vi "numpy_fft_fftfreq.vi"() -> ()   [LabVIEW 2020]
panel:
  out "n*d":fxp<+,32,16>
  out "val":fxp<+,64,48>
  out "f":fxp<+/-,32,16>[](array[numeric])
  out "Numeric":i32
  in  "s (sample rate)":fxp<+,16,16>
  out "p 2":fxp<+/-,32,32>[](array[numeric])
  out "output array":fxp<+/-,32,32>[](array[numeric])
  out "p1":fxp<+/-,32,32>[](array[numeric])
  out "N":fxp<+/-,18,17>
  in  "n":fxp<+,16,16>
  # "n=512"
  # "s=51200"
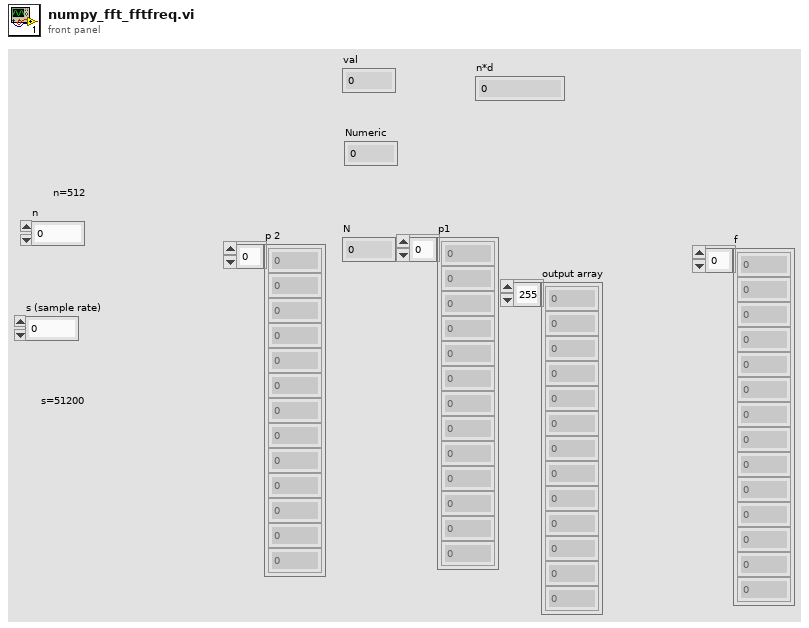
[diagram p1: front panel]
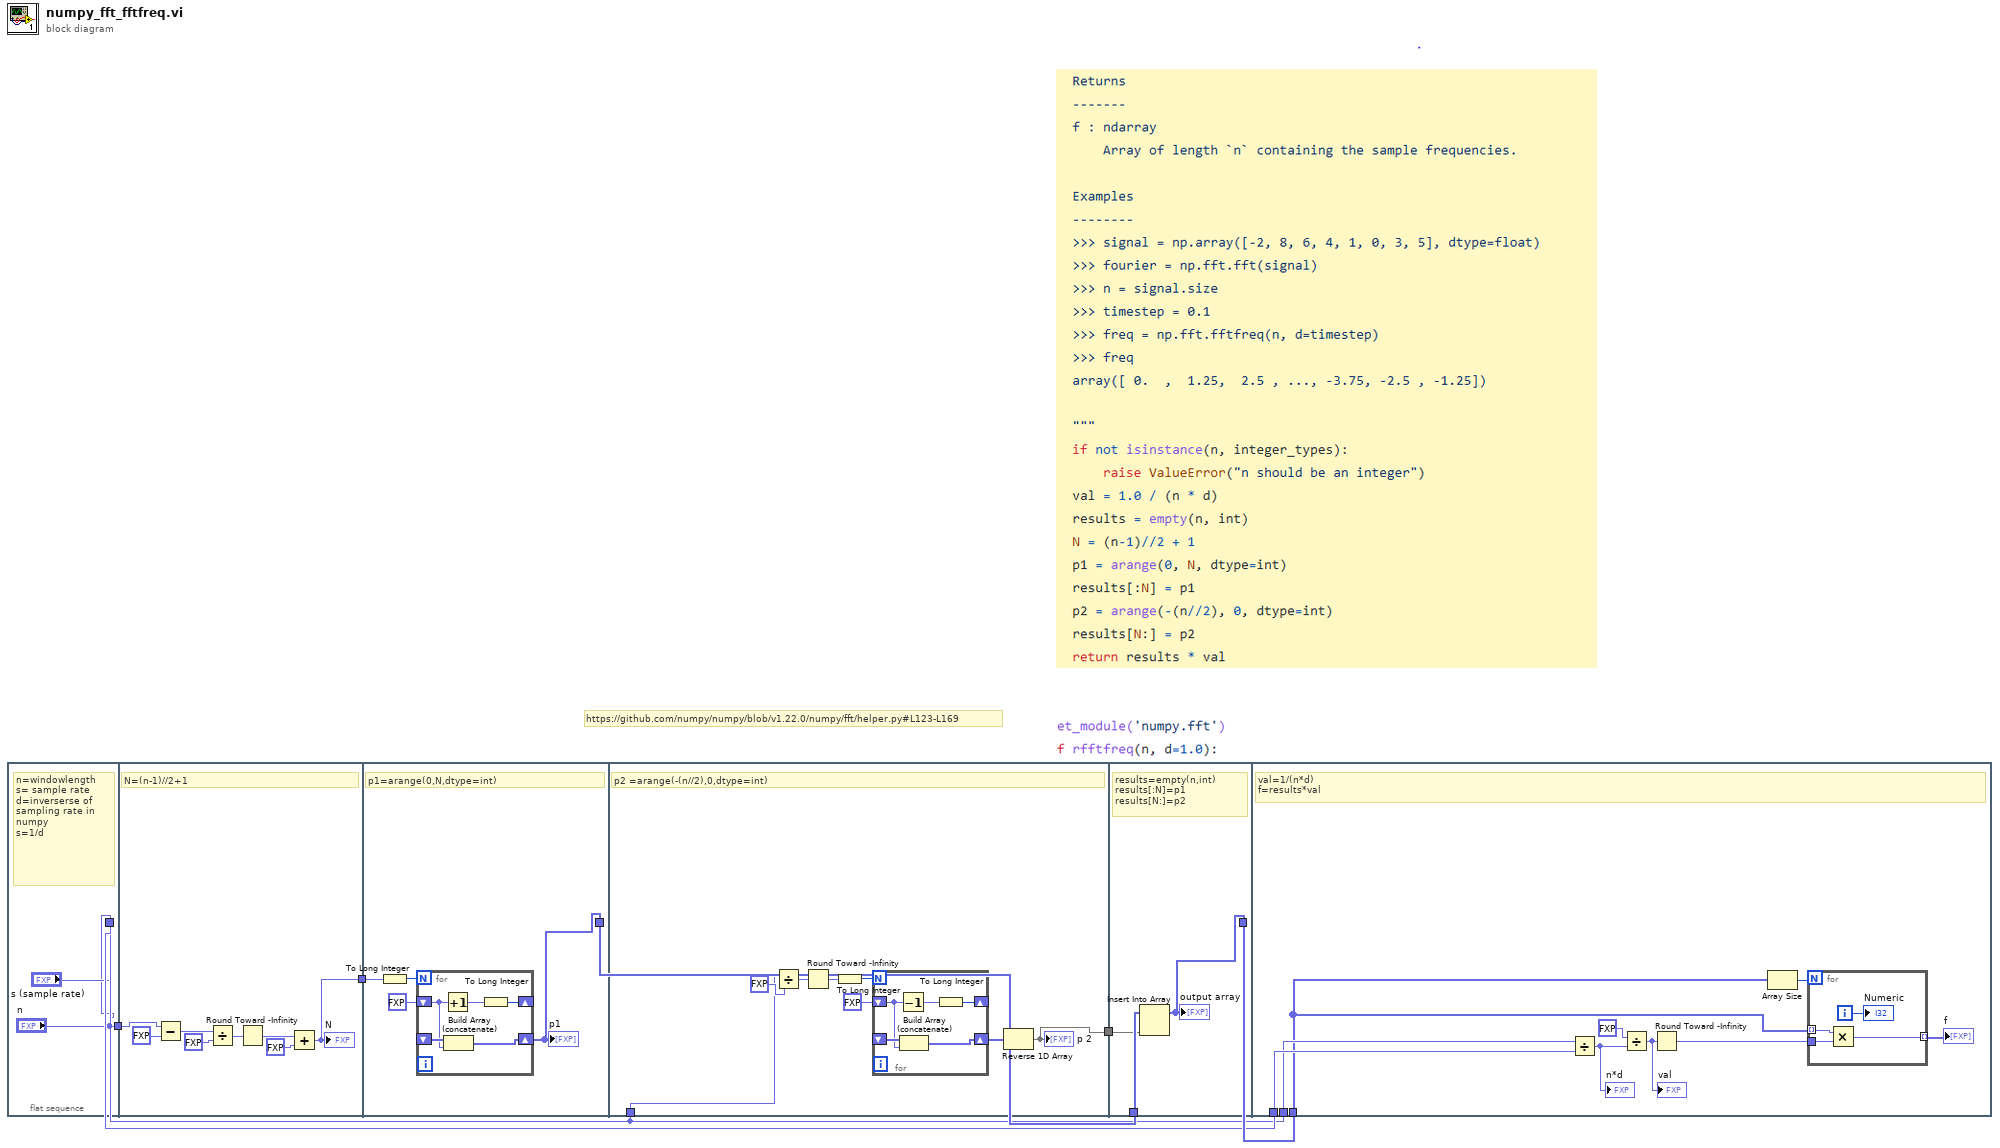
[diagram p0: block diagram]
diagram:
  # "https://github.com/numpy/numpy/blob/v1.22.0/numpy/fft/helper.py#L123-L169"
  n1 = flat-sequence {
    tunnel: ["n"] -> w3
    tunnel: ["s (sample rate)"] -> w2
    tunnel: ["n"] -> w1
    tunnel: [w11] -> w7
    tunnel: w3 -> [w10]
    tunnel: w7 -> [w20]
    tunnel: [w18] -> w6
    tunnel: w1 -> [w28]
    tunnel: [w27] -> w5
    tunnel: w6 -> [w42]
    tunnel: w5 -> [w41]
    tunnel: [w40] -> w4
    tunnel: w2 -> [w46]
    tunnel: w1 -> [w45]
    tunnel: w4 -> [w44]
    frame #0 {
      # "n=windowlength\ns= sample rate\nd=inverserse of sampling rate in numpy\ns=1/d"
    }
    frame #1 {
      # "N=(n-1)//2+1"
      n2 = Subtract(x=w10, y=fxp<+,1,1> 1.0) -> (x-y=w15:fxp<+/-,17,17>)
      n3 = Divide(x=w15, y=fxp<+,1,2> 2.0) -> (x/y=w16:fxp<+/-,18,16>)
      n4 = Round Toward -Infinity(1:w16) -> (0:w17:fxp<+/-,16,16>)
      n5 = Add(x=w17, y=fxp<+,1,1> 1.0) -> (x+y=w11:fxp<+/-,18,17>)
      "N" <- w11
    }
    frame #2 {
      # "p1=arange(0,N,dtype=int)"
      n6 = To Long Integer(number=w20) -> (32bit integer=w21:i32)
      n7 = for {
        N: w21 -> [_]
        shift-right: [w22] -> _
        shift-left: fxp<+,1,1> 0.0 -> [w24]
        shift-right: [w25] -> w18
        shift-left: _ -> [w26]
        n8 = Increment(x=w24) -> (x+1=w23:fxp<+/-,33,33>)
        n9 = Build Array (concatenate)(w26, w24) -> (w25:fxp<+/-,32,32>[])
        n10 = To Long Integer(number=w23) -> (32bit integer=w22:i32)
      }
      "p1" <- w18
    }
    frame #3 {
      # "p2 =arange(-(n//2),0,dtype=int)"
      n11 = Divide(x=w28, y=fxp<+,1,2> 2.0) -> (x/y=w31:fxp<+,17,15>)
      n12 = Round Toward -Infinity(1:w31) -> (0:w33:fxp<+,15,15>)
      n13 = To Long Integer(number=w33) -> (32bit integer=w32:i32)
      n14 = for {
        N: w32 -> [_]
        shift-right: [w35] -> _
        shift-left: fxp<+,1,1> 0.0 -> [w37]
        shift-right: [w38] -> w34
        shift-left: _ -> [w39]
        n15 = Decrement(x=w37) -> (x-1=w36:fxp<+/-,33,33>)
        n16 = Build Array (concatenate)(w39, w37) -> (w38:fxp<+/-,32,32>[])
        n17 = To Long Integer(number=w36) -> (32bit integer=w35:i32)
      }
      n18 = Reverse 1D Array(array=w34) -> (reversed array=w27:fxp<+/-,32,32>[])
      "p 2" <- w27
    }
    frame #4 {
      # "results=empty(n,int)\nresults[:N]=p1\nresults[N:]=p2"
      n19 = Insert Into Array(array=w42, new element=w41) -> (w40:fxp<+/-,32,32>[])  [unwired: 1 in]
      "output array" <- w40
    }
    frame #5 {
      # "val=1/(n*d)\nf=results*val"
      n20 = Divide(x=w45, y=w46) -> (x/y=w49:fxp<+,32,16>)
      "n*d" <- w49
      n21 = Divide(x=fxp<+,32,32> 1.0, y=w49) -> (x/y=w50:fxp<+,64,48>)
      "val" <- w50
      n22 = Round Toward -Infinity(1:w50) -> (0:w51:fxp<+,48,48>)
      n23 = Array Size(array=w44) -> (size(s)=w48:i32)
      n24 = for {
        N: w48 -> [_]
        tunnel: w44 -> [w55] mode=indexing
        tunnel: w51 -> [w54]
        tunnel: [w53] -> w47 mode=indexing
        i -> [w52]
        n25 = Multiply(x=w55, y=w54) -> (x*y=w53:fxp<+/-,32,16>)
        "Numeric" <- w52
      }
      "f" <- w47
    }
  }
